vi "Calc Power.vi"(8 "MCU_I_s_q":dbl, 9 "MCU_U_s_q":dbl, 10 "MCU_U_s_d":dbl, 11 "MCU_I_s_d":dbl) -> (3 "Power":dbl format="%#_g W")   [LabVIEW 2024, in "HSU MCU V2 CFG.lvclass"]
uses:
  HSU MCU V2 CFG.lvclass
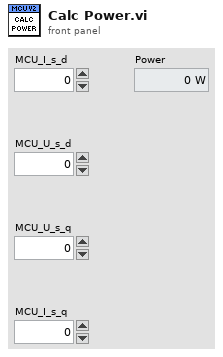
[diagram p1: front panel]
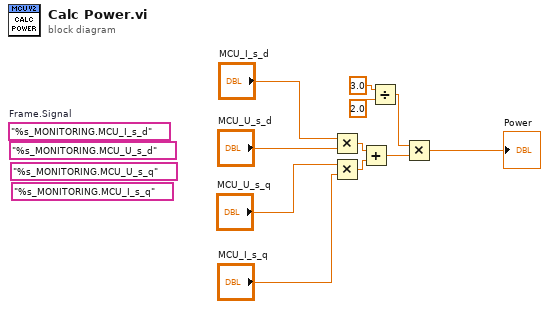
[diagram p0: block diagram]
diagram:
  (unwired) "%s_MONITORING.MCU_I_s_q" ("Frame.Signal")
  (unwired) "%s_MONITORING.MCU_U_s_q" ("Frame.Signal")
  (unwired) "%s_MONITORING.MCU_U_s_d" ("Frame.Signal")
  (unwired) "%s_MONITORING.MCU_I_s_d"  # Frame.Signal
  n1 = Multiply(x="MCU_I_s_d", y="MCU_U_s_d") -> (x*y=w11:dbl)
  n2 = Multiply(x="MCU_U_s_q", y="MCU_I_s_q") -> (x*y=w10:dbl)
  n3 = Add(x=w11, y=w10) -> (x+y=w9:dbl)
  n4 = Divide(x=3.0, y=2.0) -> (x/y=w6:dbl)
  n5 = Multiply(x=w6, y=w9) -> (x*y=→"Power":dbl)
